vi "test variant to json array.vi"(8 "error in (no error)":errorcluster) -> (0 "error out":errorcluster)   [LabVIEW 2019, in "labview_json_tests.lvlib"]
uses:
  labview_json_tests.lvlib
  lib/labview_json.lvlib
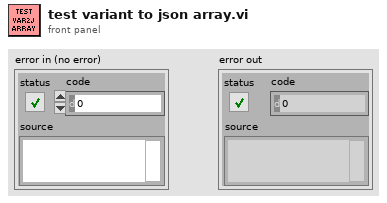
[diagram p1: front panel]
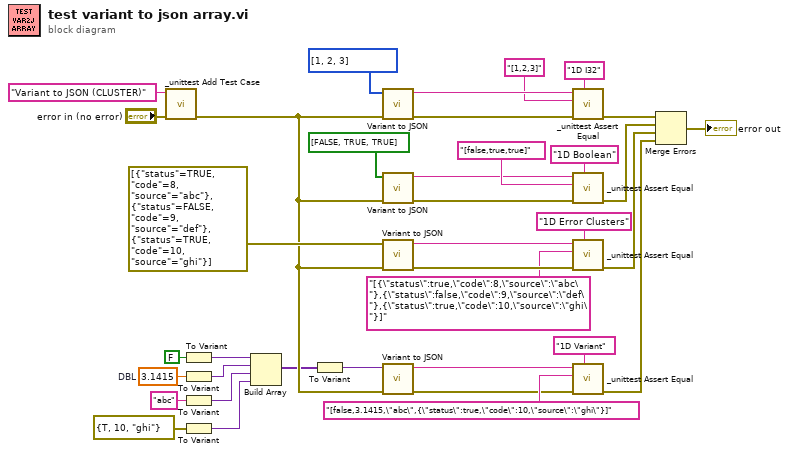
[diagram p0: block diagram]
diagram:
  w7 = 3.1415  # DBL
  n1 = call "_unittest Add Test Case.vi"("error in (no error)"="error in (no error)", "Test Case"="Variant to JSON (CLUSTER)") -> ("error out"=w11:errorcluster)  [unwired: 9 in]
  n2 = To Variant(anything=FALSE) -> (Variant=w9:variant)
  n3 = To Variant(anything=w7) -> (Variant=w6:variant)
  n4 = To Variant(anything="abc") -> (Variant=w4:variant)
  n5 = To Variant(anything=errorcluster {"status"=TRUE, "code"=10, "source"="ghi"} ("error out")) -> (Variant=w2:variant)
  n6 = Build Array(w9, w6, w4, w2) -> (w8:variant[])
  n7 = To Variant(anything=w8) -> (Variant=w1:variant)
  n8 = call "Variant to JSON.vi"("error in (no error)"=w11, "Variant in"=i32[] [1, 2, 3] ("Array")) -> ("error out"=w32:errorcluster, "JSON"=w31:string)  [unwired: 8 in]
  n9 = call "Variant to JSON.vi"("error in (no error)"=w11, "Variant in"=bool[] [FALSE, TRUE, TRUE] ("Array")) -> ("error out"=w25:errorcluster, "JSON"=w26:string)  [unwired: 8 in]
  n10 = call "Variant to JSON.vi"("error in (no error)"=w11, "Variant in"=errorcluster[] [{"status"=TRUE, "code"=8, "source"="abc"}, {"status"=FALSE, "code"=9, "source"="def"}, {"status"=TRUE, "code"=10, "source"="ghi"}]) -> ("error out"=w21:errorcluster, "JSON"=w20:string)  [unwired: 8 in]
  n11 = call "Variant to JSON.vi"("error in (no error)"=w11, "Variant in"=w1) -> ("error out"=w14:errorcluster, "JSON"=w15:string)  [unwired: 8 in]
  n12 = call "_unittest Assert Equal.vi"("Message"="1D I32", "error in (no error)"=w32, "Expected Value"="[1,2,3]", "Actual Value"=w31) -> ("error out"=w35:errorcluster)  [unwired: 7 in]
  n13 = call "_unittest Assert Equal.vi"("Message"="1D Boolean", "error in (no error)"=w25, "Expected Value"="[false,true,true]", "Actual Value"=w26) -> ("error out"=w23:errorcluster)  [unwired: 7 in]
  n14 = call "_unittest Assert Equal.vi"("Message"="1D Error Clusters", "error in (no error)"=w21, "Expected Value"="[{\"status\":true,\"code\":8,\"source\":\"abc\"},{\"status\":false,\"code\":9,\"source\":\"def\"},{\"status\":true,\"code\":10,\"source\":\"ghi\"}]", "Actual Value"=w20) -> ("error out"=w18:errorcluster)  [unwired: 7 in]
  n15 = call "_unittest Assert Equal.vi"("Message"="1D Variant", "error in (no error)"=w14, "Expected Value"="[false,3.1415,\"abc\",{\"status\":true,\"code\":10,\"source\":\"ghi\"}]", "Actual Value"=w15) -> ("error out"=w12:errorcluster)  [unwired: 7 in]
  n16 = Merge Errors(w35, w23, w18, w12) -> (→"error out":errorcluster)
